vi "Record Raw Data.vi"(8 "error in (no error)":errorcluster, 9 "Configuration Cluster":refnum<vi>, 10 "Raw Data":waveform(u8), 11 "Command":T1) -> (0 "error out":errorcluster)   [LabVIEW 2017]
uses:
  LoggingCommands.ctl
  <vilib>/Utility/sysdir.llb/System Directory Type.ctl
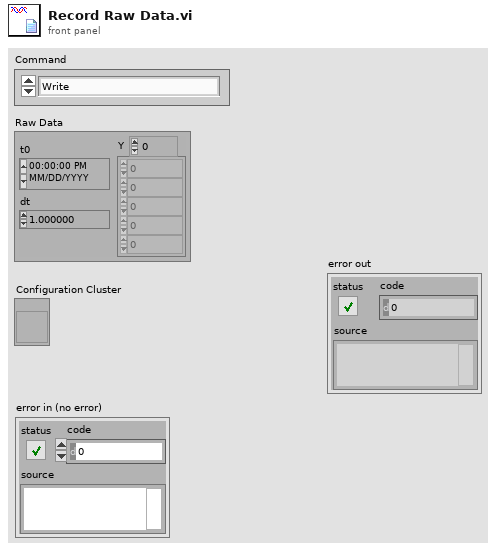
[diagram p1: front panel]
types:
  T1 = typedef "LoggingCommands.ctl" = enum16{"Write", "Close File", "Open File", "Set Channel Metadata"}
  T2 = enum16{"open", "open or create", "create or replace", "create", "open (read-only)"}
  T3 = typedef "System Directory Type.ctl" = i32
  T4 = cluster{"Center Frequency":u32, "Sample Rate (Bandwidth)":u32, "Tuner AGC Mode":bool, "AGC Mode":bool, "Manual Gain":u16, "Number of Averages":u32, "Frequency Correction":i32}
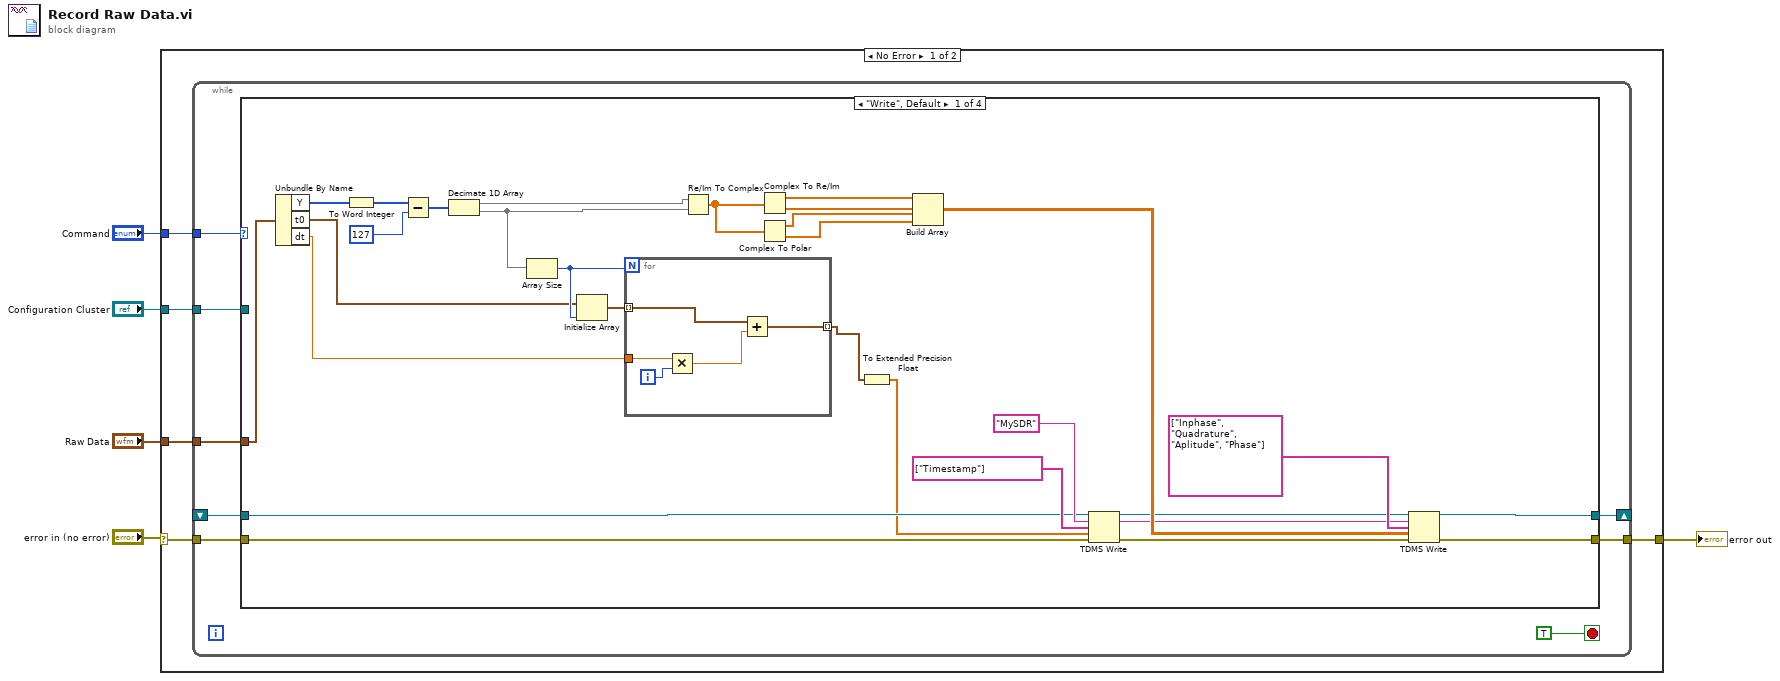
[diagram p0: block diagram]
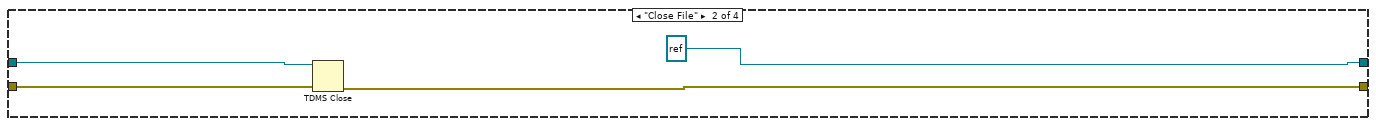
[diagram p2: hidden frame]
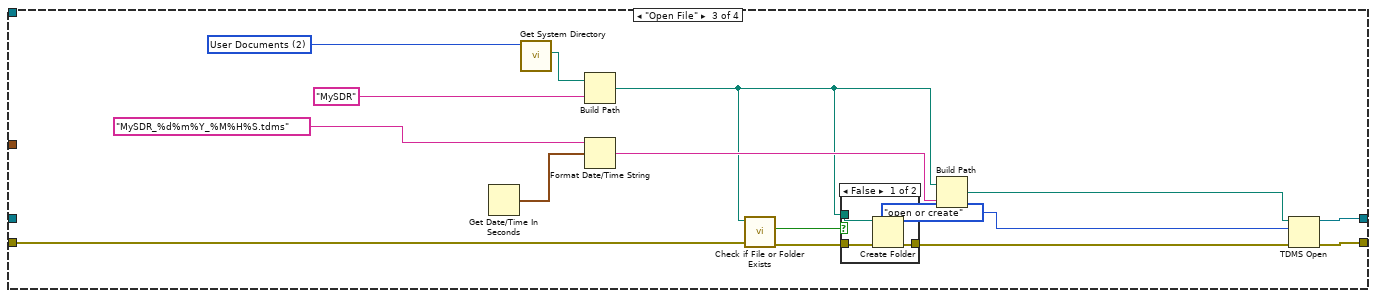
[diagram p3: hidden frame]
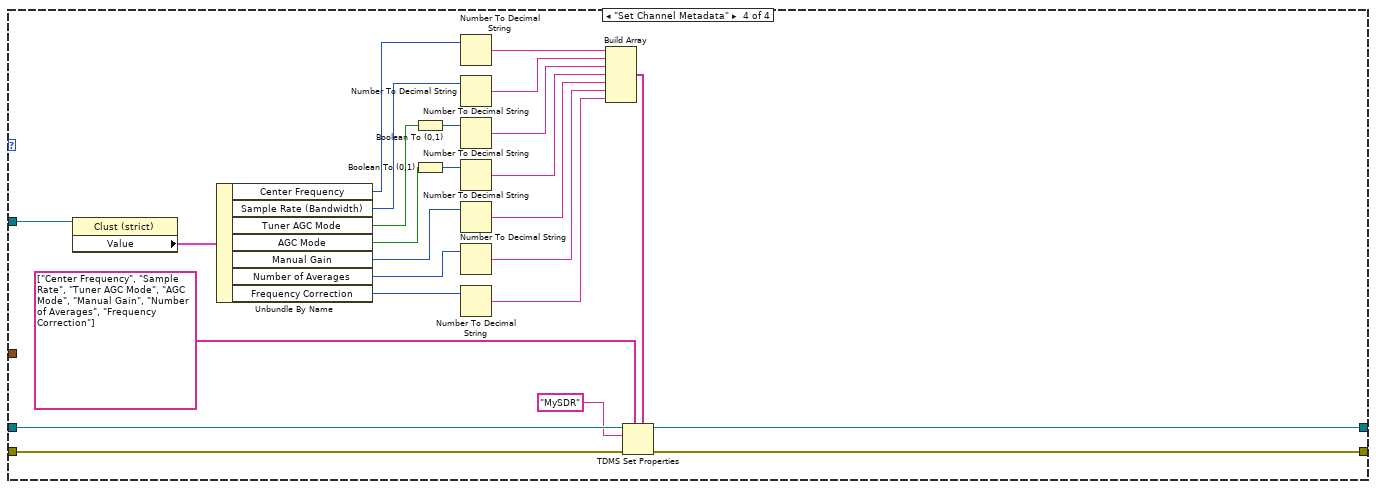
[diagram p5: hidden frame]
diagram:
  n1 = case shown="No Error" "error in (no error)" {
    selector: "error in (no error)" -> [w9 w101]
    tunnel: [w8 w101] -> w4
    tunnel: "Command" -> [w10 _]
    tunnel: "Raw Data" -> [w7 _]
    tunnel: "Configuration Cluster" -> [w6 _]
    frame No Error {
      n2 = while {
        tunnel: w10 -> [w17]
        tunnel: w9 -> [w16]
        tunnel: [w15] -> w8
        shift-right: [w14] -> _
        shift-left: _ -> [w13]
        tunnel: w7 -> [w12]
        tunnel: w6 -> [w11]
        stop <- TRUE stop-if-true
        n3 = case shown="\"Write\", Default" w17 {
          tunnel: w16 -> [w28 w56 w60 w100]
          tunnel: [w47 w55 w71 w99] -> w15
          tunnel: [w46 refnum<k34> refnum ("tdms file out") w62 w97] -> w14
          tunnel: w13 -> [w23 w54 _ w98]
          tunnel: w12 -> [w39 _ _ _]
          tunnel: w11 -> [_ _ _ w95]
          frame "Write", Default {
            n4 = Unbundle By Name(w39) -> ("Y"=w33:u8[], "t0"=w30:timestamp, "dt"=w29:dbl)
            n5 = To Word Integer(number=w33) -> (16bit integer=w38:i16[])
            n6 = Subtract(x=w38, y=i16 127) -> (x-y=w36:i16[])
            n7 = Decimate 1D Array(w36) -> (w35:i16[], w21:i16[])
            n8 = Array Size(array=w21) -> (size(s)=w32:i32)
            n9 = Initialize Array(w30, w32) -> (w31:timestamp[])
            n10 = for {
              N: w32 -> [_]
              tunnel: w31 -> [w52] mode=indexing
              tunnel: w29 -> [w50]
              tunnel: [w48] -> w20 mode=indexing
              i -> [w51]
              n11 = Multiply(x=w50, y=w51) -> (x*y=w49:dbl)
              n12 = Add(x=w52, y=w49) -> (x+y=w48:timestamp)
            }
            n13 = Re/Im To Complex(1:w21, 2:w35) -> (0:w34:cdb[])
            n14 = Complex To Re/Im(x + iy=w34) -> (x=w45:dbl[], y=w44:dbl[])
            n15 = Complex To Polar(r * e^(i*theta)=w34) -> (r=w41:dbl[], theta=w40:dbl[])
            n16 = To Extended Precision Float(1:w20) -> (0:w19:ext[])
            n17 = Build Array(w45, w44, w41, w40) -> (w43:dbl[][])
            n18 = TDMS Write(0:w23, 5:"MySDR" ("group name in (Untitled)"), 7:string[] ["Timestamp"] ("channel name(s) in (Untitled)"), 9:w19, 11:w28) -> (4:w22:refnum<k34>, 6:w25:string, 15:w27:errorcluster)  [unwired: 1 in, 1 out]
            n19 = TDMS Write(0:w22, 5:w25, 7:string[] ["Inphase", "Quadrature", "Aplitude", "Phase"] ("channel name(s) in (Untitled)"), 9:w43, 11:w27) -> (4:w46:refnum<k34>, 15:w47:errorcluster)  [unwired: 1 in, 2 out]
          }
          frame "Close File" {
            n20 = TDMS Close(8:w56, 11:w54) -> (0:w55:errorcluster)  [unwired: 1 out]
          }
          frame "Open File" {
            w70 = T3 2 items=["User Home"=0, "User Desktop"=1, "User Documents"=2, "User Application Data"=3, "User Preferences"=4, "User Temporary"=5, "Public Documents"=6, "Public Application Data"=7, "Public Preferences"=8, "Public Cache"=13, "System Core Libraries"=9, "System Installed Libraries"=10, "Application Files"=11, "Boot Volume Root"=12] ("system directory type")
            n21 = Get Date/Time In Seconds() -> (seconds since 1Jan1904=w67:timestamp)
            n22 = call <vilib>:"Get System Directory.vi"("system directory type"=w70) -> ("system directory"=w69:path)  [unwired: 10 in]
            n23 = Build Path(base path=w69, name or relative path="MySDR") -> (appended path=w57:path)
            n24 = Format Date/Time String(time format string (%c)="MySDR_%d%m%Y_%M%H%S.tdms", seconds (now)=w67) -> (date/time string=w65:string)  [unwired: 1 in]
            n25 = call <vilib>:"Check if File or Folder Exists.vi"("error in (no error)"=w60, "path"=w57) -> ("error out"=w59:errorcluster, "file or folder exists?"=w58:bool)  [unwired: 7 in, 1 out]
            n26 = case shown="False" w58 {
              tunnel: [w74 w75] -> w61
              tunnel: w59 -> [w73 w75]
              tunnel: w57 -> [w72 _]
              frame False {
                n27 = Create Folder(path (use dialog)=w72, error in=w73) -> (error out=w74:errorcluster)  [unwired: 1 in, 2 out]
              }
              frame True {
              }
            }
            n28 = Build Path(base path=w57, name or relative path=w65) -> (appended path=w64:path)
            n29 = TDMS Open(8:w61, 10:T2."open or create" ("operation (0:open)"), 11:w64) -> (0:w71:errorcluster, 3:w62:refnum<k34>)  [unwired: 4 in]
          }
          frame "Set Channel Metadata" {
            n30 = property class="Clust (strict)"(reference=w95) -> ("Value"=w94:T4)  [unwired: 1 in, 2 out]
            n31 = Unbundle By Name(w94) -> ("Center Frequency"=w93:u32, "Sample Rate (Bandwidth)"=w92:u32, "Tuner AGC Mode"=w89:bool, "AGC Mode"=w88:bool, "Manual Gain"=w85:u16, "Number of Averages"=w84:u32, "Frequency Correction"=w83:i32)
            n32 = Boolean To (0,1)(Boolean=w89) -> (0, 1=w87:i16)
            n33 = Boolean To (0,1)(Boolean=w88) -> (0, 1=w86:i16)
            n34 = Number To Decimal String(number=w93) -> (decimal integer string=w91:string)  [unwired: 1 in]
            n35 = Number To Decimal String(number=w92) -> (decimal integer string=w90:string)  [unwired: 1 in]
            n36 = Number To Decimal String(number=w87) -> (decimal integer string=w82:string)  [unwired: 1 in]
            n37 = Number To Decimal String(number=w86) -> (decimal integer string=w81:string)  [unwired: 1 in]
            n38 = Number To Decimal String(number=w85) -> (decimal integer string=w80:string)  [unwired: 1 in]
            n39 = Number To Decimal String(number=w84) -> (decimal integer string=w79:string)  [unwired: 1 in]
            n40 = Number To Decimal String(number=w83) -> (decimal integer string=w78:string)  [unwired: 1 in]
            n41 = Build Array(w91, w90, w82, w81, w80, w79, w78) -> (w77:string[])
            n42 = TDMS Set Properties(5:w77, 7:string[] ["Center Frequency", "Sample Rate", "Tuner AGC Mode", "AGC Mode", "Manual Gain", "Number of Averages", "Frequency Correction"] ("property names"), 8:w100, 10:"MySDR" ("group name"), 11:w98) -> (0:w99:errorcluster, 3:w97:refnum<k34>)  [unwired: 1 in, 2 out]
          }
        }
      }
    }
    frame Error {
    }
  }
  "error out" <- w4
